vi "SetSelectRowColor.vi"(9 "OthersRowColor":u32(colorbox)=16448250, 10 "SelectRowColor":u32(colorbox)=12369084, 11 "Table输入":refnum<vi>) -> ()   [LabVIEW 2018]
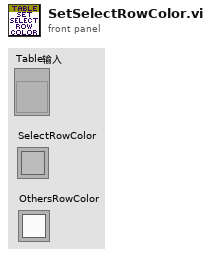
[diagram p1: front panel]
types:
  T1 = typedef "LVRowAndColumnTypeDef.ctl" = cluster{"Row":i32, "Column":i32}
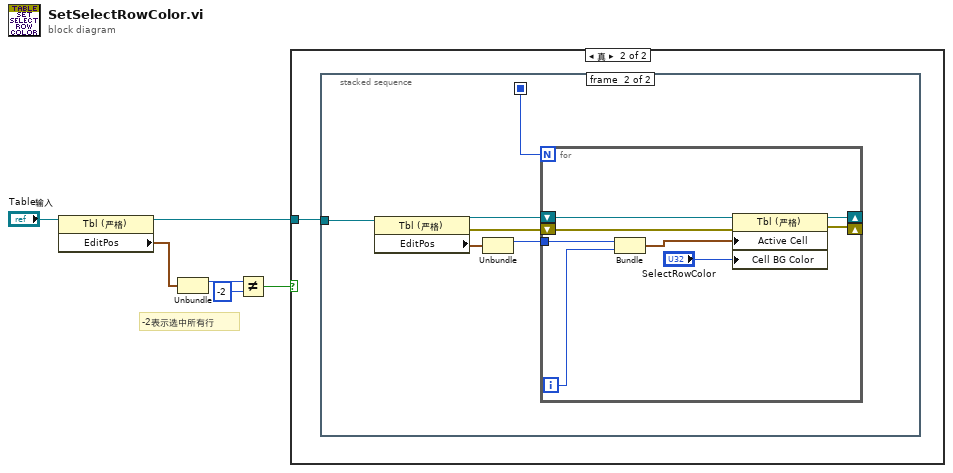
[diagram p0: block diagram]
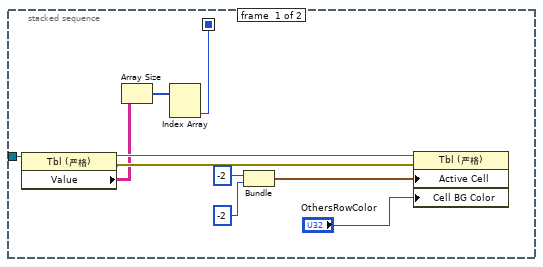
[diagram p3: hidden frame]
diagram:
  # "-2表示选中所有行"
  n1 = property class="Tbl (严格)"(reference="Table输入") -> (reference out=w5:refnum<vi>, "EditPos"=w4:T1)  [unwired: 1 in, 1 out]
  n2 = Unbundle(w4) -> ("Row"=w3:i32)  [unwired: 1 out]
  n3 = Not Equal?(x=w3, y=-2) -> (x != y?=w1:bool)
  n4 = case shown="真" w1 {
    tunnel: w5 -> [_ w7]
    frame False {
    }
    frame True {
      n5 = stacked-sequence {
        seq-local: [w12 _] -> [_ w18]
        tunnel: w7 -> [w17 w23]
        frame #0 {
          n6 = property class="Tbl (严格)"(reference=w17) -> (reference out=w16:refnum<vi>, error out=w15:errorcluster, "Value"=w14:string[][])  [unwired: 1 in]
          n7 = Array Size(array=w14) -> (size(s)=w13:i32[])
          n8 = Index Array(array=w13) -> (element #2=w12:i32)  [unwired: 2 in, 1 out]
          n9 = Bundle(-2, -2) -> (w8:cluster{i32, i32})  [unwired: 1 in]
          n10 = property class="Tbl (严格)"(reference=w16, error in=w15, "Active Cell"=w8, "Cell BG Color"="OthersRowColor") -> ()  [unwired: 2 out]
        }
        frame #1 {
          n11 = property class="Tbl (严格)"(reference=w23) -> (reference out=w21:refnum<vi>, error out=w20:errorcluster, "EditPos"=w22:T1)  [unwired: 1 in]
          n12 = Unbundle(w22) -> ("Row"=w19:i32)  [unwired: 1 out]
          n13 = for {
            N: w18 -> [_]
            tunnel: w19 -> [w28]
            shift-right: [w27] -> _
            shift-left: w21 -> [w31]
            shift-right: [w26] -> _
            shift-left: w20 -> [w30]
            i -> [w25]
            n14 = Bundle("Row"=w28, w25) -> (w29:cluster{"Row":i32, i32})  [unwired: 1 in]
            n15 = property class="Tbl (严格)"(reference=w31, error in=w30, "Active Cell"=w29, "Cell BG Color"="SelectRowColor") -> (reference out=w27:refnum<vi>, error out=w26:errorcluster)
          }
        }
      }
    }
  }
